vi "Add Data to History.vi"(6 "Check special fields? (F)":bool, 7 "Add to Undo?":bool, 8 "error in":errorcluster, 11 "Data in":T1={"Class"={"Ants"=refnum, "Layer"=refnum, "Templates"=refnum, "Icon"=refnum, "Glyph"=refnum, "Settings"=refnum, "Tools"=refnum}, "Ref"={"Add Layer"=refnum, "Remove Layer"=refnum, "Line Text"=[], "Body Text Spec"=refnum, "DNL_Font"=refnum, "glyph path str"=refnum, "templates path str"=refnum, "Arrow Up"=refnum, "Arrow Down"=refnum, "IE VI Ref"=refnum, "Glyphs tree"=refnum, "Templates tree"=refnum, "Layer Icon Text"=refnum, "Layer Template"=refnum, "Clipboard"=refnum, "BW icon in"=refnum, "Color icon in"=refnum, "Layer Clust"=refnum, "Body Text"=refnum, "DNL_Framework Templates"=refnum, "Search Templates"=refnum, "TextMarker"=refnum, "Tab Control"=refnum, "Search Glyphs"=refnum, "Line Color"=refnum, "DNL_Glyphs []"=refnum, "Fill Color"=refnum, "Tools"=refnum, "Glyphs tree"=refnum, "Icon"=refnum, "Preview"=refnum, "Ants"=refnum, "Terminals"=refnum, "menu reference"=refnum, "LayerNames"=[], "GlyphLoadAnimation"=refnum, "TemplateLoadAnimation"=refnum, "refreshGlyphs"=refnum, "refreshTemplates"=refnum}, "Support"={"AntsRect"={"left"=0, "top"=0, "right"=0, "bottom"=0}, "Mouse Move Coords"={"Horizontal"=0, "Vertical"=0}, "Mouse Down Coords"={"Horizontal"=0, "Vertical"=0}, "Temp Coord"={"Horizontal"=0, "Vertical"=0}, "Action"=enum."Default", "Edge Color"=4914962, "Fill Color"=16860, "Mouse Down?"=FALSE, "Draft Mode?"=FALSE, "Temp Icon"=bytes[3102], "CTRL Pressed"=FALSE, "Move Selection?"=FALSE, "AntsRect Orig"={"left"=0, "top"=0, "right"=0, "bottom"=0}, "Text"="", "TM Set?"=FALSE, "Mouse inside icon?"=FALSE, "Tool (old value)"=0, "Pencil Move Color"=0, "Swap Colors?"=FALSE, "Shift pressed?"=FALSE}}) -> (0 "error out":errorcluster, 3 "Data out":T1={"Class"={"Ants"=refnum, "Layer"=refnum, "Templates"=refnum, "Icon"=refnum, "Glyph"=refnum, "Settings"=refnum, "Tools"=refnum}, "Ref"={"Add Layer"=refnum, "Remove Layer"=refnum, "Line Text"=[], "Body Text Spec"=refnum, "DNL_Font"=refnum, "glyph path str"=refnum, "templates path str"=refnum, "Arrow Up"=refnum, "Arrow Down"=refnum, "IE VI Ref"=refnum, "Glyphs tree"=refnum, "Templates tree"=refnum, "Layer Icon Text"=refnum, "Layer Template"=refnum, "Clipboard"=refnum, "BW icon in"=refnum, "Color icon in"=refnum, "Layer Clust"=refnum, "Body Text"=refnum, "DNL_Framework Templates"=refnum, "Search Templates"=refnum, "TextMarker"=refnum, "Tab Control"=refnum, "Search Glyphs"=refnum, "Line Color"=refnum, "DNL_Glyphs []"=refnum, "Fill Color"=refnum, "Tools"=refnum, "Glyphs tree"=refnum, "Icon"=refnum, "Preview"=refnum, "Ants"=refnum, "Terminals"=refnum, "menu reference"=refnum, "LayerNames"=[], "GlyphLoadAnimation"=refnum, "TemplateLoadAnimation"=refnum, "refreshGlyphs"=refnum, "refreshTemplates"=refnum}, "Support"={"AntsRect"={"left"=0, "top"=0, "right"=0, "bottom"=0}, "Mouse Move Coords"={"Horizontal"=0, "Vertical"=0}, "Mouse Down Coords"={"Horizontal"=0, "Vertical"=0}, "Temp Coord"={"Horizontal"=0, "Vertical"=0}, "Action"=enum."Default", "Edge Color"=4914962, "Fill Color"=16860, "Mouse Down?"=FALSE, "Draft Mode?"=FALSE, "Temp Icon"=bytes[3102], "CTRL Pressed"=FALSE, "Move Selection?"=FALSE, "AntsRect Orig"={"left"=0, "top"=0, "right"=0, "bottom"=0}, "Text"="", "TM Set?"=FALSE, "Mouse inside icon?"=FALSE, "Tool (old value)"=0, "Pencil Move Color"=0, "Swap Colors?"=FALSE, "Shift pressed?"=FALSE}})   [LabVIEW 2021]
uses:
  <resource>/plugins/NIIconEditor/Controls/IE Data.ctl
  <resource>/plugins/NIIconEditor/Class/Ants/Ants.lvclass
  <resource>/plugins/NIIconEditor/Class/FakedArray/FakedArray.lvclass
  <resource>/plugins/NIIconEditor/Class/Icon Library/Glyph.lvclass
  <resource>/plugins/NIIconEditor/Class/Settings/Settings.lvclass
  <resource>/plugins/NIIconEditor/Class/Tools/Tools Paint.lvclass
  <vilib>/LabVIEW Icon API/lv_icon/Classes/Icon/Icon.lvclass
  <resource>/plugins/NIIconEditor/Controls/IE Classes.ctl
  <resource>/plugins/NIIconEditor/Controls/References Cluster.ctl
  <resource>/plugins/NIIconEditor/Controls/SupportClass.ctl
  <vilib>/Utility/miscctls.llb/LVPoint32TypeDef.ctl
  <resource>/plugins/NIIconEditor/Controls/SupportClass_Action.ctl
  <vilib>/LabVIEW Icon API/lv_icon/Controls/IEColor.ctl
  <resource>/plugins/NIIconEditor/Controls/Undo Redo Action.ctl
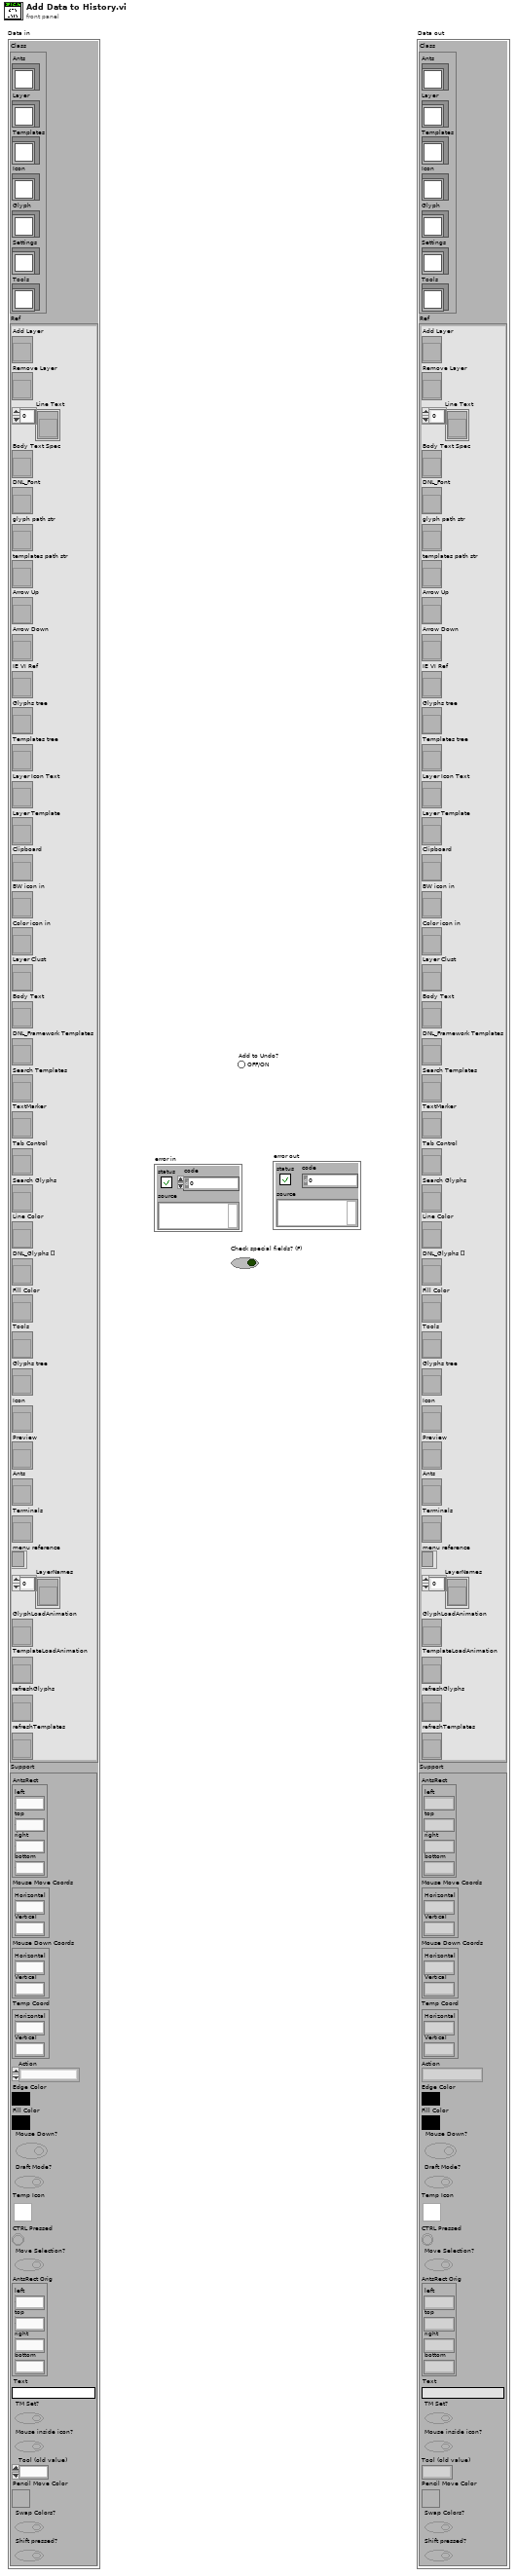
[diagram p1: front panel]
types:
  T1 = typedef "IE Data.ctl" = cluster{"Class":T2, "Ref":T3, "Support":T4}
  T2 = typedef "IE Classes.ctl" = cluster{"Ants":refnum<class "Ants.lvclass">, "Layer":refnum<class "FakedArray.lvclass">, "Templates":refnum<class "FakedArray.lvclass">, "Icon":refnum<class "Icon.lvclass">, "Glyph":refnum<class "Glyph.lvclass">, "Settings":refnum<class "Settings.lvclass">, "Tools":refnum<class "Tools Paint.lvclass">}
  T3 = typedef "References Cluster.ctl" = cluster{"Add Layer":refnum<vi>, "Remove Layer":refnum<vi>, "Line Text":refnum<vi>[], "Body Text Spec":refnum<vi>, "DNL_Font":refnum<vi>, "glyph path str":refnum<vi>, "templates path str":refnum<vi>, "Arrow Up":refnum<vi>, "Arrow Down":refnum<vi>, "IE VI Ref":refnum<vi>, "Glyphs tree":refnum<vi>, "Templates tree":refnum<vi>, "Layer Icon Text":refnum<vi>, "Layer Template":refnum<vi>, "Clipboard":refnum<vi>, "BW icon in":refnum<vi>, "Color icon in":refnum<vi>, "Layer Clust":refnum<vi>, "Body Text":refnum<vi>, "DNL_Framework Templates":refnum<vi>, "Search Templates":refnum<vi>, "TextMarker":refnum<vi>, "Tab Control":refnum<vi>, "Search Glyphs":refnum<vi>, "Line Color":refnum<vi>, "DNL_Glyphs []":refnum<vi>, "Fill Color":refnum<vi>, "Tools":refnum<vi>, "Glyphs tree":refnum<vi>, "Icon":refnum<vi>, "Preview":refnum<vi>, "Ants":refnum<vi>, "Terminals":refnum<vi>, "menu reference":refnum<k9>, "LayerNames":refnum<vi>[], "GlyphLoadAnimation":refnum<vi>, "TemplateLoadAnimation":refnum<vi>, "refreshGlyphs":refnum<vi>, "refreshTemplates":refnum<vi>}
  T4 = typedef "SupportClass.ctl" = cluster{"AntsRect":cluster{"left":i16, "top":i16, "right":i16, "bottom":i16}, "Mouse Move Coords":T5, "Mouse Down Coords":T5, "Temp Coord":T5, "Action":T6, "Edge Color":T7, "Fill Color":T7, "Mouse Down?":bool, "Draft Mode?":bool, "Temp Icon":picture, "CTRL Pressed":bool, "Move Selection?":bool, "AntsRect Orig":cluster{"left":i16, "top":i16, "right":i16, "bottom":i16}, "Text":string, "TM Set?":bool, "Mouse inside icon?":bool, "Tool (old value)":u32, "Pencil Move Color":u32, "Swap Colors?":bool, "Shift pressed?":bool}
  T5 = typedef "LVPoint32TypeDef.ctl" = cluster{"Horizontal":i32, "Vertical":i32}
  T6 = typedef "SupportClass_Action.ctl" = enum16{"Default", "Move Selection", "Glyph Library", "Tool"}
  T7 = typedef "IEColor.ctl" = u32
  T8 = typedef "Undo Redo Action.ctl" = enum16{"Init", "Add", "Redo", "Undo", "Undo Preview"}
  T9 = cluster{"LayerIcon":picture, "LayerName":string, "Opacity":u8, "Visibility?":bool}
  T10 = typedef "Font.ctl" = string
  T11 = typedef "Alignment.ctl" = u16
  T12 = typedef "Font Size.ctl" = u8
  T13 = cluster{"Line 1 text":string, "Line 2 text":string, "Line 3 text":string, "Line 4 text":string, "Line 1 color":u32, "Line 2 color":u32, "Line 3 color":u32, "Line 4 color":u32, "Body Text Spec":cluster{"DNL_Font":T10, "Alignment":T11, "Size":T12}, "Center text vertically":bool, "Capitalize Text":bool}
  T14 = typedef "Graphic.ctl" = cluster{"Rectangle":cluster{"left":i16, "top":i16, "right":i16, "bottom":i16}, "Path":path, "Image":picture, "Filter":string, "FileName":string}
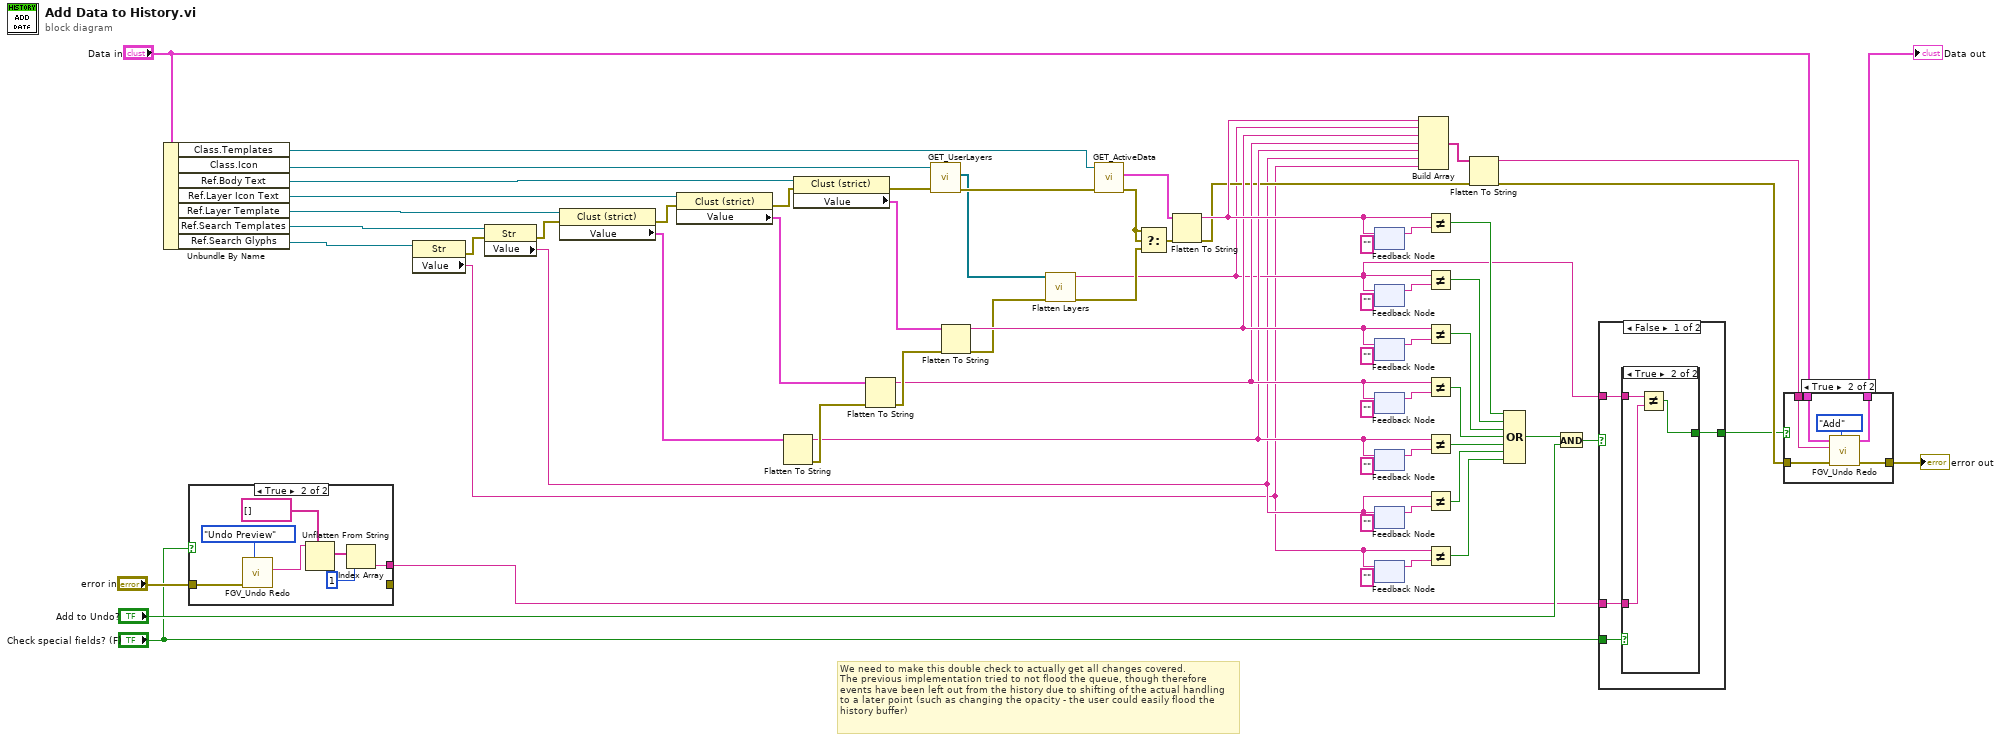
[diagram p0: block diagram]
diagram:
  # "We need to make this double check to actually get all changes covered.\nThe previous implementation tried to not flood the queue, though therefore\nevents have been left out from the history due to shifting of the actual handling\nto a later point (such as changing the opacity - the user could easily flood the\nhistory buffer)"
  n1 = Unbundle By Name("Data in") -> ("Class.Templates"=w27:refnum<class "FakedArray.lvclass">, "Class.Icon"=w29:refnum<class "Icon.lvclass">, "Ref.Body Text"=w66:refnum<vi>, "Ref.Layer Icon Text"=w65:refnum<vi>, "Ref.Layer Template"=w64:refnum<vi>, "Ref.Search Templates"=w12:refnum<vi>, "Ref.Search Glyphs"=w9:refnum<vi>)
  n2 = case shown="True" "Check special fields? (F)" {
    tunnel: "error in" -> [w67 w74]
    tunnel: [w67 _] -> _
    tunnel: [_ w69] -> w19
    frame False {
    }
    frame True {
      n3 = call <resource>:"FGV_Undo Redo.vi"("Action"=Undo_Redo_Action."Undo Preview", "error in (no error)"=w74) -> ("Data out"=w71:string)  [unwired: 3 in, 6 out]
      n4 = Unflatten From String(type=string[] [] ("appended array"), binary string=w71) -> (value=w70:string[])  [unwired: 3 in, 2 out]
      n5 = Index Array(array=w70, index=1) -> (element=w69:string)
    }
  }
  n6 = property class="Str"(reference=w9) -> (error out=w10:errorcluster, "Value"=w1:string)  [unwired: 1 in, 1 out]
  n7 = property class="Str"(reference=w12, error in=w10) -> (error out=w11:errorcluster, "Value"=w2:string)  [unwired: 1 out]
  n8 = property class="Clust (strict)"(reference=w64, error in=w11) -> (error out=w57:errorcluster, "Value"=w58:T9)  [unwired: 1 out]
  n9 = property class="Clust (strict)"(reference=w65, error in=w57) -> (error out=w52:errorcluster, "Value"=w56:T9)  [unwired: 1 out]
  n10 = Flatten To String(anything=w58) -> (data string=w34:string, error out=w51:errorcluster)  [unwired: 1 in, 3 out]
  n11 = property class="Clust (strict)"(reference=w66, error in=w52) -> (error out=w28:errorcluster, "Value"=w53:T13)  [unwired: 1 out]
  n12 = Flatten To String(anything=w56, error in (no error)=w51) -> (data string=w35:string, error out=w50:errorcluster)  [unwired: 3 out]
  n13 = call-dynamic "GET_UserLayers.vi"("error in (no error)"=w28, "Icon.lvclass in"=w29) -> ("error out"=w26:errorcluster, "All Layers"=w13:refnum<class "Layer.lvclass">[])  [unwired: 8 out]
  n14 = Flatten To String(anything=w53, error in (no error)=w50) -> (data string=w36:string, error out=w16:errorcluster)  [unwired: 3 out]
  n15 = call <resource>:"Flatten Layers.vi"("Error In"=w16, "Layers"=w13) -> ("Error Out"=w15:errorcluster, "String"=w14:string)  [unwired: 8 in]
  n16 = call-dynamic "GET_ActiveData.vi"("error in (no error)"=w26, "FakedArray in"=w27) -> ("error out"=w39:errorcluster, "Path & Icon"=w45:T14)  [unwired: 8 out]
  n17 = Select(t=w39, s=w39, f=w15) -> (s? t:f=w38:errorcluster)
  n18 = Flatten To String(anything=w45, error in (no error)=w38) -> (data string=w37:string, error out=w31:errorcluster)  [unwired: 3 out]
  n19 = feedback-in #1(w37) -> ()
  n20 = feedback #1("" ("data string")) -> (w47:string)
  n21 = feedback-in #2(w14) -> ()
  n22 = feedback #2("" ("data string")) -> (w48:string)
  n23 = feedback-in #3(w36) -> ()
  n24 = feedback #3("" ("data string")) -> (w55:string)
  n25 = feedback-in #4(w35) -> ()
  n26 = feedback #4("" ("data string")) -> (w59:string)
  n27 = feedback-in #5(w34) -> ()
  n28 = feedback #5("" ("data string")) -> (w62:string)
  n29 = feedback #6("" ("data string")) -> (w7:string)
  n30 = feedback-in #6(w2) -> ()
  n31 = feedback #7("" ("data string")) -> (w6:string)
  n32 = feedback-in #7(w1) -> ()
  n33 = Build Array(w37, w14, w36, w35, w34, w2, w1) -> (w33:string[])
  n34 = Not Equal?(x=w37, y=w47) -> (x != y?=w40:bool)
  n35 = Not Equal?(x=w14, y=w48) -> (x != y?=w41:bool)
  n36 = Not Equal?(x=w36, y=w55) -> (x != y?=w42:bool)
  n37 = Not Equal?(x=w35, y=w59) -> (x != y?=w43:bool)
  n38 = Not Equal?(x=w34, y=w62) -> (x != y?=w44:bool)
  n39 = Not Equal?(x=w2, y=w7) -> (x != y?=w4:bool)
  n40 = Not Equal?(x=w1, y=w6) -> (x != y?=w3:bool)
  n41 = Flatten To String(anything=w33, error in (no error)=w31) -> (data string=w21:string, error out=w32:errorcluster)  [unwired: 3 out]
  n42 = Compound Arithmetic op=OR(w40, w41, w42, w43, w44, w4, w3) -> (w23:bool)
  n43 = And(x=w23, y="Add to Undo?") -> (x .and. y?=w18:bool)
  n44 = case shown="False" w18 {
    selector: w18 -> [_ w82]
    tunnel: [w76 w82] -> w22
    tunnel: w14 -> [w78 _]
    tunnel: w19 -> [w77 _]
    tunnel: "Check special fields? (F)" -> [w75 _]
    frame False {
      n45 = case shown="True" w75 {
        tunnel: w78 -> [_ w81]
        tunnel: w77 -> [_ w80]
        tunnel: [_ w79] -> w76
        frame False {
        }
        frame True {
          n46 = Not Equal?(x=w81, y=w80) -> (x != y?=w79:bool)
        }
      }
    }
    frame True {
    }
  }
  n47 = case shown="True" w22 {
    tunnel: [w84 w89] -> w63
    tunnel: w32 -> [w84 w88]
    tunnel: w21 -> [_ w87]
    tunnel: "Data in" -> [w83 w86]
    tunnel: [w83 w85] -> w30
    frame False {
    }
    frame True {
      n48 = call <resource>:"FGV_Undo Redo.vi"("Action"=Undo_Redo_Action."Add", "error in (no error)"=w88, 10:"Data in"=w87, 11:"Data in"=w86) -> ("error out"=w89:errorcluster, "Data out"=w85:T1)  [unwired: 1 in, 5 out]
    }
  }
  "error out" <- w63
  "Data out" <- w30
